vi "kalmanFilterForBalls.vi"(0 "Use Observation":bool=TRUE, 1 "intervalo":dbl=1.0, 2 "Pk-1|k-1":T1, 3 "z_k":T1, 5 "error in (no error)":errorcluster, 6 "x_k-1|k-1":T1=[[0.0, 0.0, 0.0], [0.0, 0.0, 0.0], [0.0, 0.0, 0.0]]) -> (14 "Pk|k out":T1, 16 "x_k|k out":T1, 17 "Conf":dbl, 19 "error out":errorcluster)   [LabVIEW 2023, in "Vision.lvclass"]
uses:
  Vision.lvclass
  <vilib>/Analysis/Matrix/Datatypes/RealMatrix.ctl
  <vilib>/Analysis/_algsub.llb/Real Matrix Norm.vi
  <vilib>/Analysis/NI_AALPro.lvlib
  <vilib>/Analysis/Matrix/NI_Matrix.lvlib
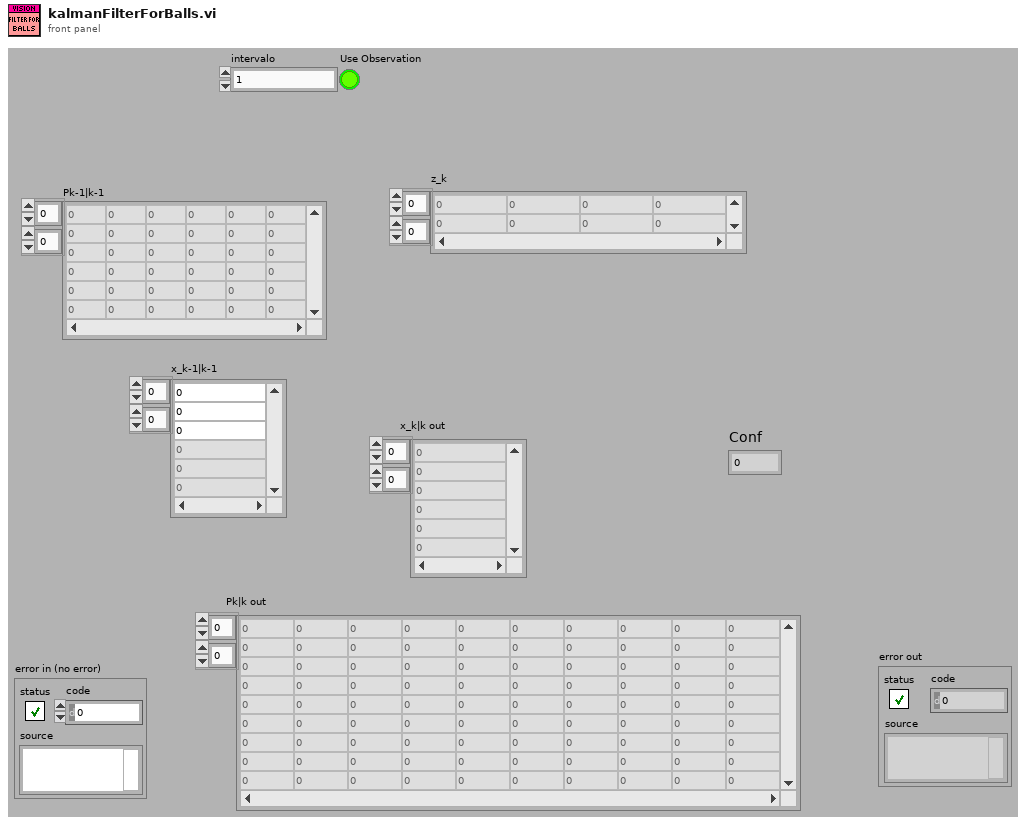
[diagram p1: front panel]
types:
  T1 = typedef "NI_Matrix.lvlib/RealMatrix.ctl" = dbl[][]
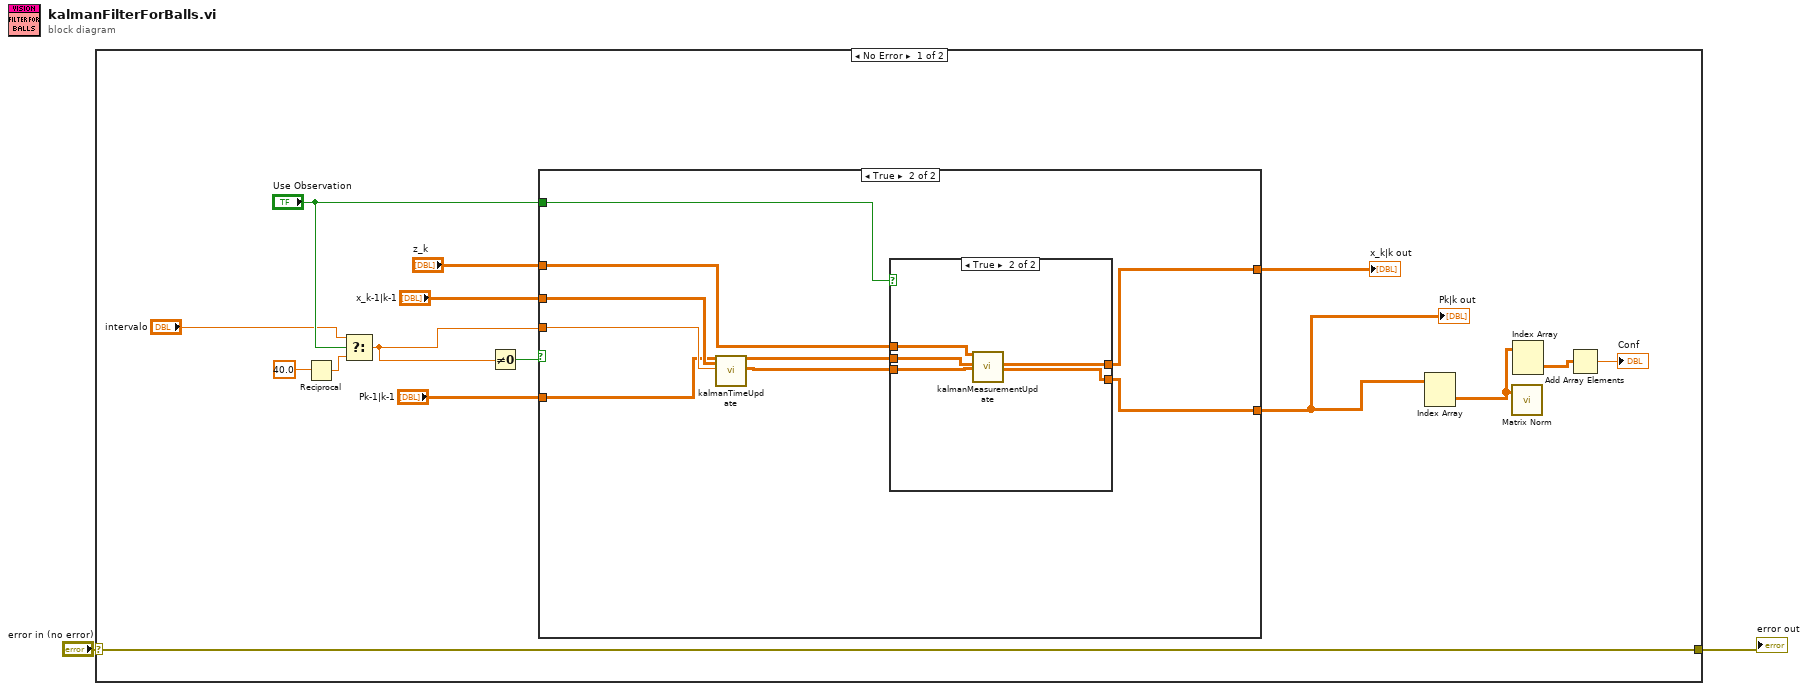
[diagram p0: block diagram]
diagram:
  n1 = case shown="No Error" "error in (no error)" {
    selector: "error in (no error)" -> [w17 w36]
    tunnel: [w17 w36] -> w1
    frame No Error {
      n2 = Reciprocal(x=40.0) -> (1/x=w7:dbl)
      n3 = Select(t="intervalo", s="Use Observation", f=w7) -> (s? t:f=w6:dbl)
      n4 = Not Equal To 0?(x=w6) -> (x != 0?=w3:bool)
      n5 = case shown="True" w3 {
        tunnel: w6 -> [_ w27]
        tunnel: [w19 w21] -> w11
        tunnel: "Pk-1|k-1" -> [w18 w25]
        tunnel: "x_k-1|k-1" -> [w19 w26]
        tunnel: [w18 w20] -> w14
        tunnel: "z_k" -> [_ w22]
        tunnel: "Use Observation" -> [_ w28]
        frame False {
        }
        frame True {
          n6 = call "kalmanTimeUpdate.vi"("Pk-1|k-1"=w25, "x_k-1|k-1"=w26, "intervalo"=w27) -> ("x_k|k out"=w24:T1, "Pk|k out"=w23:T1)  [unwired: 14 in, 1 out]
          n7 = case shown="True" w28 {
            tunnel: w24 -> [w30 w35]
            tunnel: w23 -> [w29 w34]
            tunnel: w22 -> [_ w33]
            tunnel: [w30 w32] -> w21
            tunnel: [w29 w31] -> w20
            frame False {
            }
            frame True {
              n8 = call "kalmanMeasurementUpdate.vi"("z_k"=w33, "x_k-1|k-1"=w35, "Pk-1|k-1"=w34) -> ("x_k-1|k-1 out"=w32:T1, "Pk-1|k-1 out"=w31:T1)  [unwired: 14 in, 1 out]
            }
          }
        }
      }
      "Pk|k out" <- w14
      "x_k|k out" <- w11
      n9 = Index Array(array=w14) -> (element=w13:T1)  [unwired: 2 in]
      n10 = call-poly <vilib>:"Matrix Norm.vi"("Input Matrix"=w13) -> ()  [unwired: 1 in, 2 out]
      n11 = Index Array(array=w13) -> (element=w12:T1)  [unwired: 2 in]
      n12 = Add Array Elements(numeric array=w12) -> (sum=→"Conf":dbl)
    }
    frame Error {
    }
  }
  "error out" <- w1
